vi "Digital Close.vi"(8 "Error In":errorcluster, 10 "Digtal Channel":u8[](array[numeric]), 11 "LINX Resource":T1) -> (0 "Error Out":errorcluster, 3 "LINX Resource":T1)   [LabVIEW 2014, in "LMH-LINX.lvlib"]
doc: "Close the specified digital IO channels."
uses:
  LMH-LINX.lvlib
  Private/Type Defs/LINX Ref.ctl
  Private/Type Defs/Platform.ctl
  Private/Type Defs/Interface.ctl
  Private/Device/Type Defs/LINX Device Config.ctl
  Private/Device/Type Defs/TCP Config.ctl
  Private/Device/Type Defs/Channels.ctl
  Private/Type Defs/Peripheral.ctl
  <vilib>/myRIO/Instrument Drivers/Onboard IO/DIO/DIO.lvlib
  Private/myRIO/myRIO.lvlib
  Private/Device/Device.lvlib
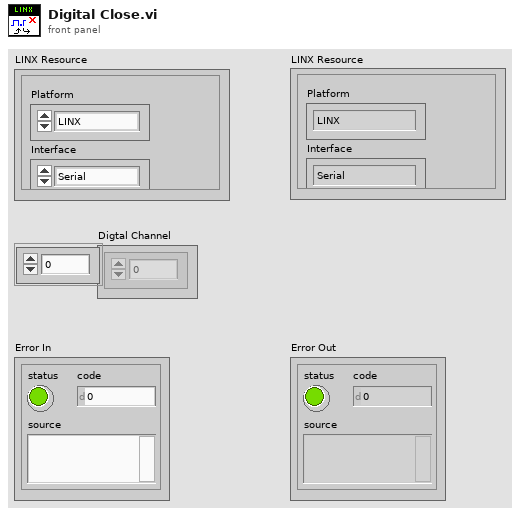
[diagram p1: front panel]
types:
  T1 = typedef "LMH-LINX.lvlib/LINX Ref.ctl" = cluster{"Platform":T2, "Interface":T3, "LINX Device Config":T4}
  T2 = typedef "LMH-LINX.lvlib/Platform.ctl" = enum16{"LINX", "myRIO"}
  T3 = typedef "LMH-LINX.lvlib/Interface.ctl" = enum16{"Serial", "TCP"}
  T4 = typedef "LMH-LINX.lvlib/Device.lvlib/LINX Device Config.ctl" = cluster{"Interface":T3, "COM Port":refnum<visa-resource-name>, "TCP Configuration":T5, "Device Family":u8, "Device ID":u8, "Device Name":string, "TCP Ref":refnum<k5>, "Channels":T6}
  T5 = typedef "LMH-LINX.lvlib/Device.lvlib/TCP Config.ctl" = cluster{"IP Address":string, "Port":u16}
  T6 = typedef "LMH-LINX.lvlib/Channels.ctl" = cluster{"DI":u8[], "DO":u8[], "AI":u8[], "AO":u8[], "PWM":u8[], "QE":u8[], "UART":u8[], "I2C 2":u8[], "SPI":u8[], "CAN":u8[], "Servo":u8[], "AI Ref (V)":dbl, "AO Ref (V)":dbl, "AO Resolution (Bits)":u8}
  T7 = typedef "LMH-LINX.lvlib/Peripheral.ctl" = enum8{"DI", "DO", "AI", "AO", "PWM", "QE", "UART", "I2C", "SPI", "CAN", "Servo"}
  T8 = typedef "DIO.lvlib/DIO Reference.ctl" = cluster{"myRIO Reference":T9, "DIO Channels List":T13}
  T9 = typedef "myRIO Generic Hardware Reference.ctl" = cluster{"myRIO Model":T10, "myRIO Hardware Reference":T11}
  T10 = typedef "Hardware Version Enum.ctl" = enum16{"Unknown", "myRIO-1900", "myRIO-1950"}
  T11 = typedef "myRIO v1.0 Reference.ctl" = cluster{"Generic FPGA Reference":T12, "Allow multiple opens":bool}
  T12 = typedef "Generic FPGA Reference.ctl" = refnum<k20>
  T13 = typedef "DIO Channels List.ctl" = T14[]
  T14 = typedef "DIO Channels Enum.ctl" = enum16{"Not Connected", "C/DIO0", "C/DIO1", "C/DIO2", "C/DIO3", "C/DIO4", "C/DIO5", "C/DIO6", "C/DIO7", "A/DIO0", "A/DIO1", "A/DIO2", "A/DIO3", "A/DIO4", "A/DIO5", "A/DIO6", "A/DIO7", "A/DIO8", "A/DIO9", "A/DIO10", "A/DIO11", "A/DIO12", "A/DIO13", "A/DIO14", "A/DIO15", "B/DIO0", "B/DIO1", "B/DIO2", "B/DIO3", "B/DIO4", "B/DIO5", "B/DIO6", "B/DIO7", "B/DIO8", "B/DIO9", "B/DIO10", "B/DIO11", "B/DIO12", "B/DIO13", "B/DIO14", "B/DIO15", "LED0", "LED1", "LED2", "LED3", "Button0"}
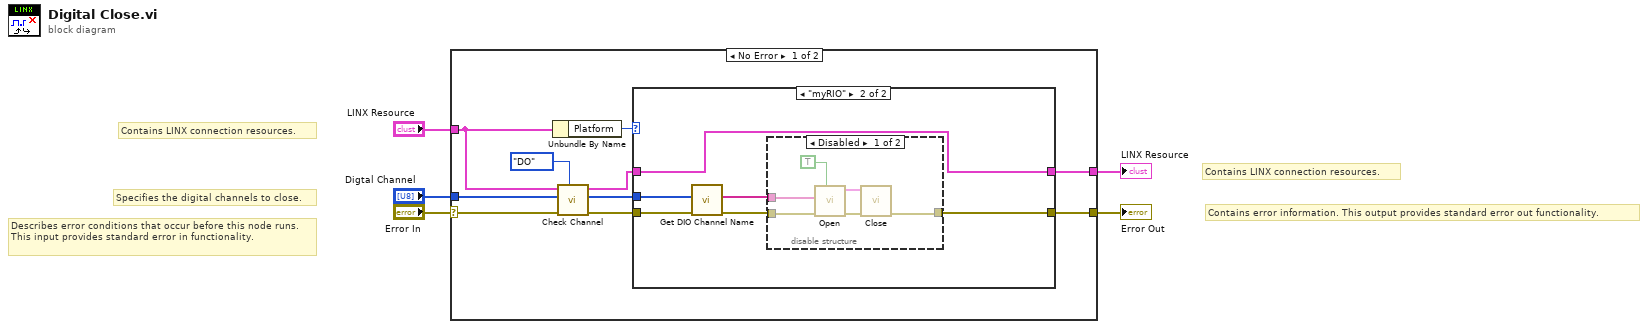
[diagram p0: block diagram]
diagram:
  # "Specifies the digital channels to close."
  # "Contains LINX connection resources."
  # "Contains error information. This output provides standard error out functionality."
  # "Contains LINX connection resources."
  # "Describes error conditions that occur before this node runs. This input provides standard error in functionality."
  n1 = case shown="No Error" "Error In" {
    selector: "Error In" -> [w6 w32]
    tunnel: [w14 w32] -> w5
    tunnel: [w13 w31] -> w4
    tunnel: "Digtal Channel" -> [w7 _]
    tunnel: "LINX Resource" -> [w8 w31]
    frame No Error {
      n2 = Unbundle By Name(w8) -> ("Platform"=w15:T2)
      n3 = call "Check Channel.vi"("Peripheral"=Peripheral."DO", "Error In"=w6, "Channels"=w7, "LINX Resource"=w8) -> ("Error Out"=w10:errorcluster, "Channels"=w11:u8[], "LINX Resource"=w9:T1)  [unwired: 5 in]
      n4 = case shown="\"myRIO\"" w15 {
        tunnel: w10 -> [w17 w22]
        tunnel: [w17 w19] -> w14
        tunnel: w11 -> [_ w23]
        tunnel: [w16 w18] -> w13
        tunnel: w9 -> [w16 w18]
        frame "LINX", Default {
          # "!!! Send Close Command (Some LINX Devices Might Have A Use For This)"
        }
        frame "myRIO" {
          n5 = call "Get DIO Channel Name.vi"("Error In"=w22, "DIO Channel Nums"=w23) -> ("Error Out"=w20:errorcluster, "DIO Channels"=w21:string[])  [unwired: 8 in]
          n6 = disable-structure shown="Disabled" {
            disable-tunnel: w21 -> [w26 _]
            disable-tunnel: w20 -> [w25 w30]
            disable-tunnel: [w24 w30] -> w19
            frame Disabled {
              n7 = call <vilib>:"Open.vi"("Allow multiple opens?"=TRUE, "error in (no error)"=w25, "Channel Names"=w26) -> ("error out"=w29:errorcluster, "DIO Ref Out"=w28:T8)  [unwired: 7 in]
              n8 = call <vilib>:"Close.vi"("error in (no error)"=w29, "DIO Ref In"=w28) -> ("error out"=w24:errorcluster)  [unwired: 9 in]
            }
            frame Enabled {
              # "myRIO Support Not Installed"
            }
          }
        }
      }
    }
    frame Error {
    }
  }
  "Error Out" <- w5
  "LINX Resource" <- w4
